vi "Cfg from FP.vi"(8 "error in (no error)":errorcluster, 11 "Monitor Controller in":refnum<class "Monitor Controller.lvclass">) -> (0 "error out":errorcluster, 3 "Monitor Controller out":refnum<class "Monitor Controller.lvclass">)   [LabVIEW 2016, in "Monitor Controller.lvclass"]
uses:
  Monitor Controller.lvclass
  C:/github/Measure_core/da Base/Template Module.lvclass
  Monitor Controller.lvclass/Monitor Controller.ctl
  Measurements/Timer Messages/Write Period Msg/Write Period Msg.lvclass/Write Period Msg.ctl
  <vilib>/ActorFramework/Message Enqueuer/Message Enqueuer.lvclass/Message Enqueuer.ctl
  Template Module/Template Module.lvclass/Template Module.ctl
  Template Module/Write Repeat times.vi
  <vilib>/ActorFramework/Message Enqueuer/Enqueue.vi
  Measurements/Timer Messages/Write Period Msg/Write Period Msg.lvclass
  C:/Program Files/National Instruments/LabVIEW 2016/vi.lib/ActorFramework/Message/Message.lvclass
  Read Monitor controller configuration.vi
  <vilib>/ActorFramework/Message Priority Queue/Priority Enqueue.vi
  Process Controller/Process Controller.lvclass
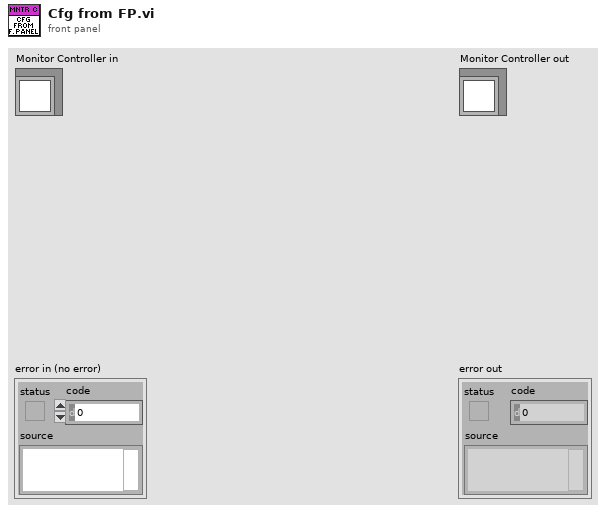
[diagram p1: front panel]
types:
  T1 = typedef "Monitor Controller Configuration.ctl" = cluster{"Period":dbl, "Repeat times":i32, "Open plot":bool, "File defragment period":dbl}
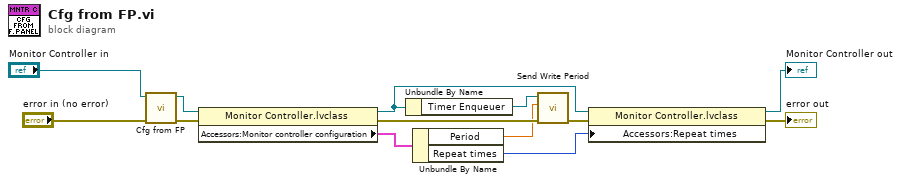
[diagram p0: block diagram]
diagram:
  n1 = call-parent "Cfg from FP.vi"("error in (no error)"="error in (no error)", "Measure Object in"="Monitor Controller in") -> ("error out"=w4:errorcluster, "Measure Object out"=w6:refnum<class "Monitor Controller.lvclass">)  [unwired: 8 in]
  n2 = property class="Monitor Controller.lvclass"(reference=w6, error in=w4) -> (reference out=w2:refnum<class "Monitor Controller.lvclass">, error out=w10:errorcluster, "Accessors:Monitor controller configuration"=w7:T1)
  n3 = Unbundle By Name(w2) -> ("Timer Enqueuer"=w1:refnum<class "Message Enqueuer.lvclass">)
  n4 = Unbundle By Name(w7) -> ("Period"=w9:dbl, "Repeat times"=w8:i32)
  n5 = call "Send Write Period.vi"("error in (no error)"=w10, "Period"=w9, "Message Enqueuer"=w1) -> ("error out"=w11:errorcluster)  [unwired: 7 in, 1 out]
  n6 = property class="Monitor Controller.lvclass"(reference=w2, error in=w11, "Accessors:Repeat times"=w8) -> (reference out=→"Monitor Controller out":refnum<class "Monitor Controller.lvclass">, error out=→"error out":errorcluster)
